vi "Setup UI.vi"(8 "error in (no error)":errorcluster, 10 "Set UI to input? (F)":bool, 11 "Photon Counter \nwith LCD Reader in":refnum<class "Photon Counter with LCD Reader.lvclass">) -> (0 "error out":errorcluster, 3 "Photon Counter \nwith LCD Reader out":refnum<class "Photon Counter with LCD Reader.lvclass">)   [LabVIEW 2017, in "Photon Counter with LCD Reader.lvclass"]
doc: "Setup UI constructs an object -- populates its member fields -- from a front panel the user can see. The VI should be as simple as possible so that a UI loop can poll it continuously for updates. \n\nThe VI is designed to be used as a subPanel within another VI. Wire true to \"Set UI to input\" only on the first call, just after inserting this VI into a subPanel, to populate its controls with the class's current values.\n\nSetup UI is distinct from the class constructor. Class constructors are not polymorphic, yet configure dialogs need to configure objects without knowing their type -- and polymorphism is the necessary solution. Thus, Setup UI is a polymorphic class constructor. This continously polled \"Setup UI\" concept is a kludge: a better idea would be an XControl, but those require a steeper learning curve."
uses:
  Photon Counter with LCD Reader.lvclass
  Photon Counter with LCD Reader.lvclass/Photon Counter with LCD Reader.ctl
panel:
  in  "Send first pt to PC":bool
  in  "Count Time":dbl[unit]=1.0 format="%#_4g"
  in  "Gate B %":dbl=0.5 min=0.0 max=1.0 step=0.01 format="%_2g"
  in  "Gate A %":dbl=0.5 min=0.0 max=1.0 step=0.01 format="%_2g"
  in  "Trigger Frequency":dbl[unit]=42076.2
  in  "LCD track the scan independent variable?":bool
  # "Photon Counter\nwith LCD Setup"
  # "(PEM = 42.0762 kHz)"
  # "Gates will be centered at T/4 and 3T/4"
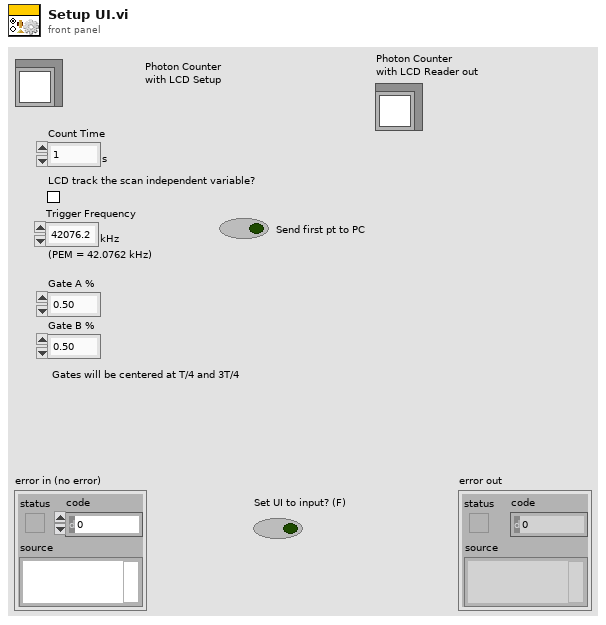
[diagram p1: front panel]
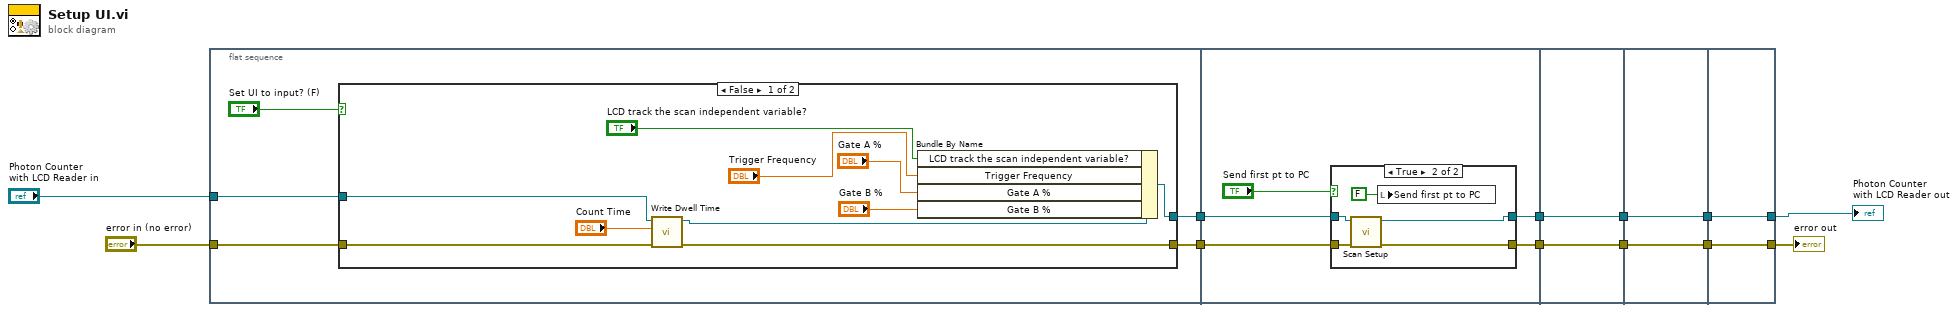
[diagram p0: block diagram]
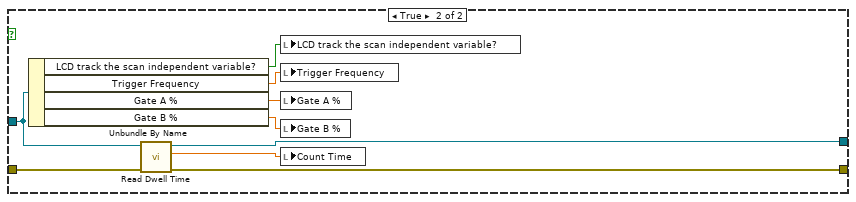
[diagram p2: hidden frame]
diagram:
  n1 = flat-sequence {
    tunnel: [w13] -> w8
    tunnel: "Photon Counter \nwith LCD Reader in" -> [w14]
    tunnel: [w15] -> w2
    tunnel: "error in (no error)" -> [w16]
    tunnel: [w39] -> w9
    tunnel: w8 -> [w40]
    tunnel: [w37] -> w3
    tunnel: w2 -> [w38]
    tunnel: [w50] -> w10
    tunnel: w9 -> [w50]
    tunnel: [w49] -> w4
    tunnel: w3 -> [w49]
    tunnel: [w52] -> w11
    tunnel: w10 -> [w52]
    tunnel: [w51] -> w5
    tunnel: w4 -> [w51]
    tunnel: [w54] -> w12
    tunnel: w11 -> [w54]
    tunnel: [w53] -> w6
    tunnel: w5 -> [w53]
    frame #0 {
      n2 = case shown="False" "Set UI to input? (F)" {
        tunnel: w14 -> [w22 w32]
        tunnel: w16 -> [w20 w31]
        tunnel: [w19 w30] -> w15
        tunnel: [w23 w29] -> w13
        frame False {
          n3 = call-dynamic "Write Dwell Time.vi"("error in (no error)"=w20, "Dwell Time"="Count Time", "Reader.lvclass in"=w22) -> ("error out"=w19:errorcluster, "Reader.lvclass out"=w21:refnum<class "Photon Counter with LCD Reader.lvclass">)  [unwired: 7 out]
          n4 = Bundle By Name(cluster=w21, "LCD track the scan independent variable?"="LCD track the scan independent variable?", "Trigger Frequency"="Trigger Frequency", "Gate A %"="Gate A %", "Gate B %"="Gate B %") -> (w23:refnum<class "Photon Counter with LCD Reader.lvclass">)
        }
        frame True {
          n5 = Unbundle By Name(w32) -> ("LCD track the scan independent variable?"=w36:bool, "Trigger Frequency"=w35:dbl[unit], "Gate A %"=w34:dbl, "Gate B %"=w33:dbl)
          n6 = call-dynamic "Read Dwell Time.vi"("error in (no error)"=w31, "Reader.lvclass in"=w32) -> ("error out"=w30:errorcluster, "Dwell Time"=w28:dbl[unit], "Reader.lvclass out"=w29:refnum<class "Photon Counter with LCD Reader.lvclass">)  [unwired: 7 out]
          n7 = local write "LCD track the scan independent variable?"(w36) -> ()
          n8 = local write "Trigger Frequency"(w35) -> ()
          n9 = local write "Gate A %"(w34) -> ()
          n10 = local write "Gate B %"(w33) -> ()
          n11 = local write "Count Time"(w28) -> ()
        }
      }
    }
    frame #1 {
      n12 = case shown="True" "Send first pt to PC" {
        tunnel: w40 -> [w43 w47]
        tunnel: [w43 w46] -> w39
        tunnel: w38 -> [w42 w45]
        tunnel: [w42 w44] -> w37
        frame False {
        }
        frame True {
          n13 = call-dynamic "Scan Setup.vi"("error in (no error)"=w45, "Photon Counter with LCD Reader in"=w47) -> ("error out"=w44:errorcluster, "Photon Counter with LCD Reader out"=w46:refnum<class "Photon Counter with LCD Reader.lvclass">)  [unwired: 8 in]
          n14 = local write "Send first pt to PC"(FALSE ("Send first pt to PC")) -> ()
        }
      }
    }
    frame #2 {
    }
    frame #3 {
    }
    frame #4 {
    }
  }
  "error out" <- w6
  "Photon Counter \nwith LCD Reader out" <- w12
